vi "for_debugs.vi"() -> ()   [LabVIEW 2015]
uses:
  convertors/typedefs/BSONelement.ctl
  convertors/typedefs/dataType.ctl
  data_cluster.ctl
  convertors/typedefs/binaryData_cluster.ctl
  convertors/typedefs/arraySettings_cluster.ctl
  <vilib>/addons/_JKI.lib/Serialization/JSON/JKI JSON Serialization.lvlib
  convertors/BSON_convertors_Library.lvlib
panel:
  out "source data":T1={"int1"=1, "int2"=2, "SS1"={"int11"=11, "int22"=22}, "SS2"={"int33"=33, "int44"=44, "LLL"={"int1"=1, "int2"=2, "int11"=11, "int22"=22}}, "dblArray"=[111.1, 112.2, 113.3, 114.0, 115.0, 116.0, 117.0, 118.0, 119.0, 120.0], "stringData"="", "U64Array"=[5555, 5556, 5557, 5558, 5559, 5560, 5561]}
  in  "Tab Control":T2(tab)
  out "JSON String":string
  out "to_BSON_error out":errorcluster
  out "BSONdocArrayAsBin":u8[](array[numeric]) format="%02x"
  out "BSONdocArrayAsArray":u8[](array[numeric]) format="%02x"
  out "to_BSON_error out 2":errorcluster
  out "arrayOfElements_hiLVL_BinData":T3[](array[typedef])
  out "arrayOfElements_first_step":T3[](array[typedef])
  out "big cluster value":T3[](array[typedef])
  out "lvl2_cluster":T3[](array[typedef])
  out "arrayOfElements_hiLVL_arrays":T3[](array[typedef])
  out "diff names (error)":T5
  out "bindata error 5001 (error)":errorcluster
  out "diff names with array (error)":T5
  out "array error 5001 (error)":errorcluster
  out "strictData from bin":T1
  out "strictData error out1":errorcluster
  out "strictData from array":T1
  out "strictData error out2":errorcluster
  out "more elements from array":T6={"int1"=1, "int2"=2, "SS1"={"int11"=11, "int22"=22}, "SS2"={"int33"=33, "int44"=44, "LLL"={"int1"=1, "int2"=2, "int11"=11, "int22"=22}}, "dblArray"=[111.0, 112.0, 113.0, 114.0, 115.0, 116.0, 117.0, 118.0, 119.0, 120.0], "U64Array"=[5555, 5556, 5557, 5558, 5559, 5560, 5561], "int88"=0, "stringData"=""}
  out "more elements from byte error out":errorcluster
  out "more elements from array error out":errorcluster
  out "more elements from bite":T6={"int1"=1, "int2"=2, "SS1"={"int11"=11, "int22"=22}, "SS2"={"int33"=33, "int44"=44, "LLL"={"int1"=1, "int2"=2, "int11"=11, "int22"=22}}, "dblArray"=[111.0, 112.0, 113.0, 114.0, 115.0, 116.0, 117.0, 118.0, 119.0, 120.0], "U64Array"=[5555, 5556, 5557, 5558, 5559, 5560, 5561], "int88"=0, "stringData"=""}
  out "Less elements from array 2":T7={"int1"=1, "int2"=2, "SS1"={"int11"=11, "int22"=22}, "SS2"={"int33"=33, "int44"=44, "LLL"={"int1"=1, "int2"=2, "int11"=11, "int22"=22}}, "dblArray"=[5555.0, 5556.0, 5557.0, 5558.0, 5559.0, 5560.0, 5561.0], "stringData"=""}
  out "Less elements from binary as binArray error out":errorcluster
  out "Less elements from binary as binArray":T8={"int1"=1, "int2"=2, "SS1"={"int11"=11, "int22"=22}, "SS2"={"int33"=33, "int44"=44, "LLL"={"int1"=1, "int2"=2, "int11"=11, "int22"=22}}, "U64Array"=[], "stringData"=""}
  out "Less elements from binary as binCluster error out":errorcluster
  out "Less elements from binary as binCluster":T10={"int1"=1, "int2"=2, "SS1"={"int11"=11, "int22"=22}, "SS2"={"int33"=33, "int44"=44, "LLL"={"int1"=1, "int2"=2, "int11"=11, "int22"=22}}, "dblArray"={"subType"=0, "byteArray"=[]}, "stringData"=""}
  out "Less elements from array":T11={"int1"=1, "int2"=2, "SS1"={"int11"=11, "int22"=22}, "SS2"={"int33"=33, "int44"=44, "LLL"={"int1"=1, "int2"=2, "int11"=11, "int22"=22}}, "U64Array"=[5555, 5556, 5557, 5558, 5559, 5560, 5561], "stringData"=""}
  out "Less elements from binary error out":errorcluster
  out "Less elements from array error out":errorcluster
  out "Less elements from binary":T7={"int1"=1, "int2"=2, "SS1"={"int11"=11, "int22"=22}, "SS2"={"int33"=33, "int44"=44, "LLL"={"int1"=1, "int2"=2, "int11"=11, "int22"=22}}, "dblArray"=[111.0, 112.0, 113.0, 114.0, 115.0, 116.0, 117.0, 118.0, 119.0, 120.0], "stringData"=""}
  out "Less elements from array error out 2":errorcluster
  # "This clusters have \"illegal\" elements for strict conversion"
  # "These clusters are exactly the same as in the package"
  # "These clusters have \"extra\" elements.\nOnly those that are in the package are filled"
  # "This clusters have fewer elements.\nOnly those that are present are filled. Excess data from the package is discarded"
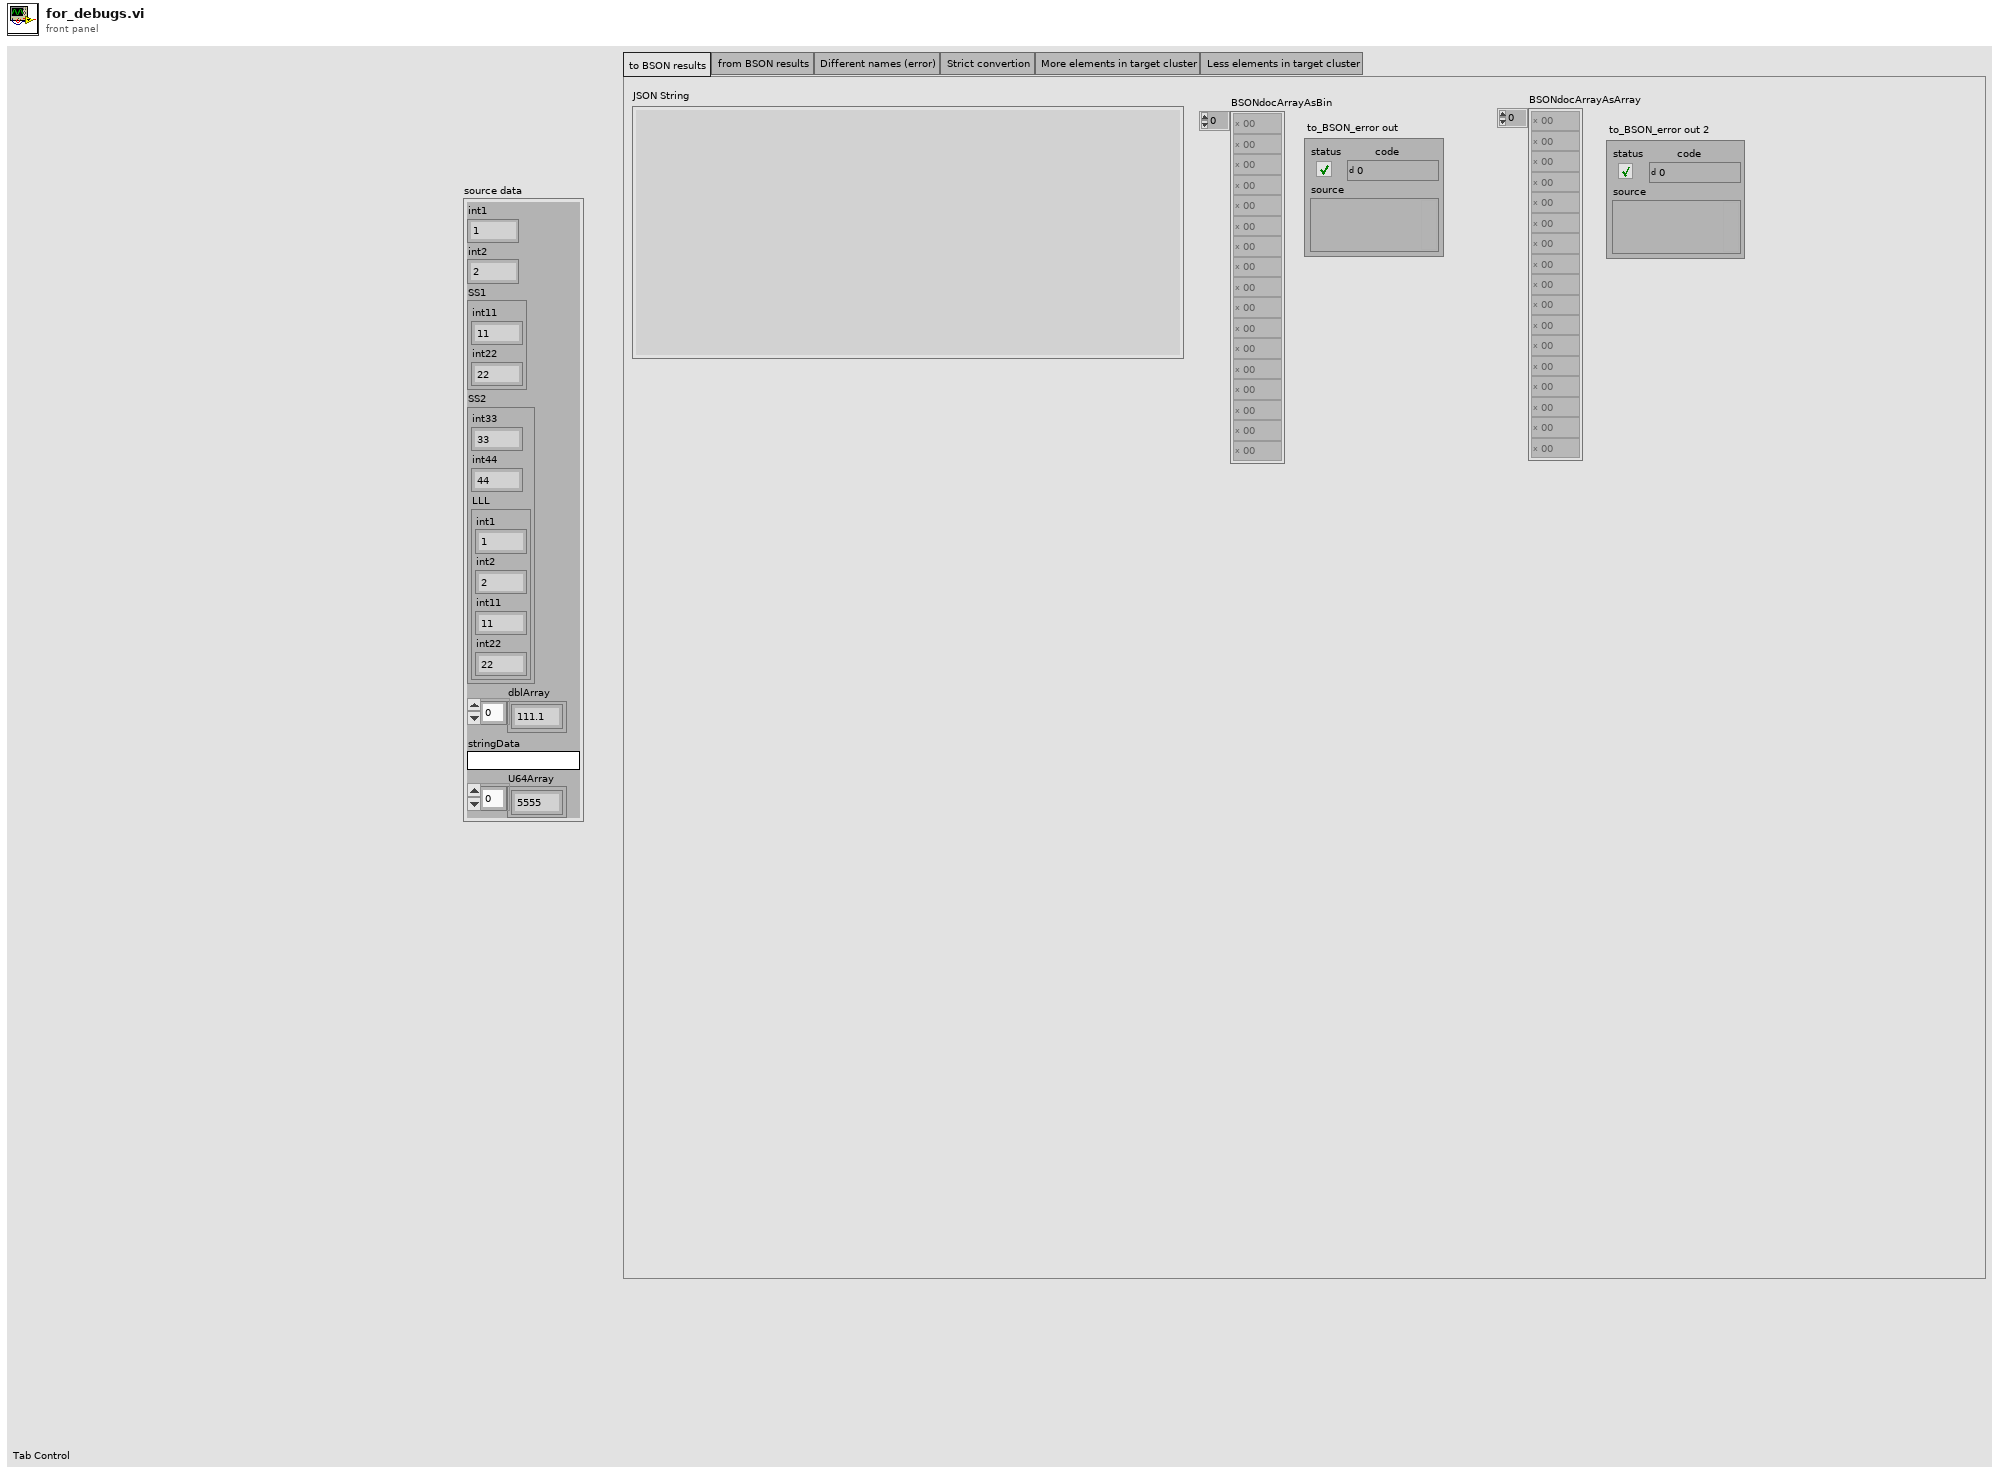
[diagram p1: front panel]
types:
  T1 = typedef "data_cluster.ctl" = cluster{"int1":i32, "int2":i32, "SS1":cluster{"int11":i32, "int22":i32}, "SS2":cluster{"int33":i32, "int44":i32, "LLL":cluster{"int1":i32, "int2":i32, "int11":i32, "int22":i32}}, "dblArray":dbl[], "stringData":string, "U64Array":u64[]}
  T2 = enum32{"to BSON results", "from BSON results", "Different names (error)", "Strict convertion", "More elements in target cluster", "Less elements in target cluster"}
  T3 = typedef "BSON_convertors_Library.lvlib/BSONelement.ctl" = cluster{"dataType":T4, "name":string, "value":variant}
  T4 = typedef "BSON_convertors_Library.lvlib/dataType.ctl" = enum8{"empty(terminator)", "double", "string", "document", "array", "binary", "Deprecated(Undefined)", "ObjectId", "boolean", "UTC datetime", "Null value", "cstring", "Deprecated(DBPointer)", "JavaScript", "Deprecated(Symbol)", "code_w_s", "int32", "uint64", "int64", "ext (decimal128)", "Min key", "Max key"}
  T5 = cluster{"int1":i32, "int2":i32, "SS1":cluster{"int11":i32, "int22":i32}, "SS2":cluster{"int3333":i32, "int44":i32, "LLL":cluster{"int1":i32, "int2":i32, "int11":i32, "int22":i32}}}
  T6 = cluster{"int1":i32, "int2":i32, "SS1":cluster{"int11":i32, "int22":i32}, "SS2":cluster{"int33":i32, "int44":i32, "LLL":cluster{"int1":i32, "int2":i32, "int11":i32, "int22":i32}}, "dblArray":dbl[], "U64Array":u64[], "int88":i32, "stringData":string}
  T7 = cluster{"int1":i32, "int2":i32, "SS1":cluster{"int11":i32, "int22":i32}, "SS2":cluster{"int33":i32, "int44":i32, "LLL":cluster{"int1":i32, "int2":i32, "int11":i32, "int22":i32}}, "dblArray":dbl[], "stringData":string}
  T8 = cluster{"int1":i32, "int2":i32, "SS1":cluster{"int11":i32, "int22":i32}, "SS2":cluster{"int33":i32, "int44":i32, "LLL":cluster{"int1":i32, "int2":i32, "int11":i32, "int22":i32}}, "U64Array":u8[], "stringData":string}
  T9 = typedef "BSON_convertors_Library.lvlib/binaryData_cluster.ctl" = cluster{"subType":u8, "byteArray":u8[]}
  T10 = cluster{"int1":i32, "int2":i32, "SS1":cluster{"int11":i32, "int22":i32}, "SS2":cluster{"int33":i32, "int44":i32, "LLL":cluster{"int1":i32, "int2":i32, "int11":i32, "int22":i32}}, "dblArray":T9, "stringData":string}
  T11 = cluster{"int1":i32, "int2":i32, "SS1":cluster{"int11":i32, "int22":i32}, "SS2":cluster{"int33":i32, "int44":i32, "LLL":cluster{"int1":i32, "int2":i32, "int11":i32, "int22":i32}}, "U64Array":u64[], "stringData":string}
  T12 = typedef "BSON_convertors_Library.lvlib/arraySettings_cluster.ctl" = cluster{"arrayAsBinData":bool, "binDataSubType":u8, "little-endian":bool}
  T13 = enum16{"open", "replace", "create", "open or create", "replace or create", "replace or create with confirmation"}
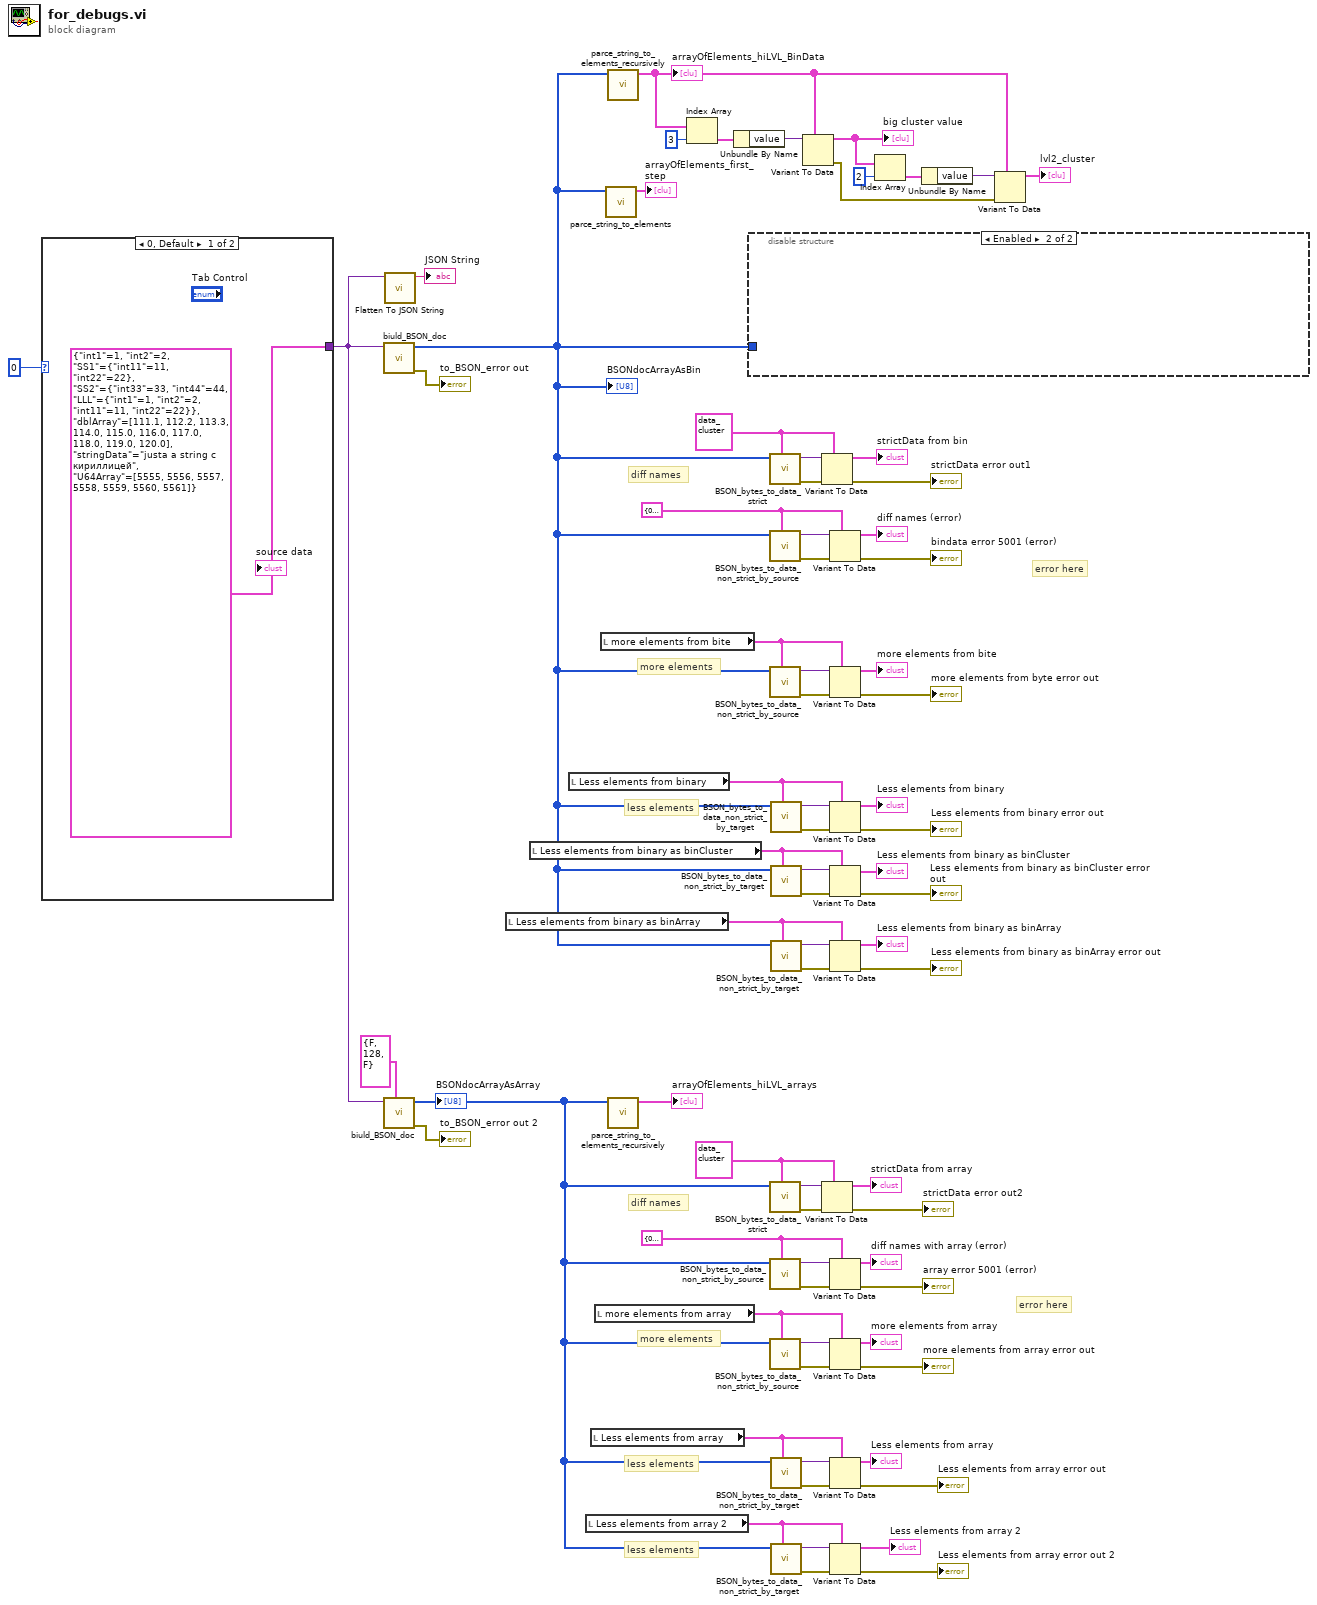
[diagram p0: block diagram]
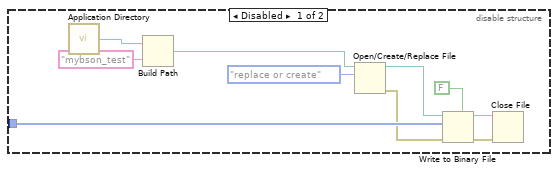
[diagram p2: hidden frame]
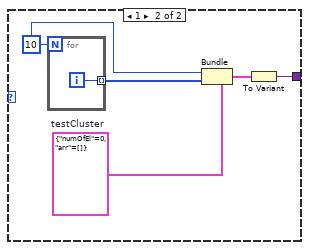
[diagram p3: hidden frame]
diagram:
  w45 = T1 {"int1"=0, "int2"=0, "SS1"={"int11"=0, "int22"=0}, "SS2"={"int33"=0, "int44"=0, "LLL"={"int1"=0, "int2"=0, "int11"=0, "int22"=0}}, "dblArray"=[], "stringData"="", "U64Array"=[]} ("LLL")
  w43 = T5 {"int1"=0, "int2"=0, "SS1"={"int11"=0, "int22"=0}, "SS2"={"int3333"=0, "int44"=0, "LLL"={"int1"=0, "int2"=0, "int11"=0, "int22"=0}}}
  w51 = T1 {"int1"=0, "int2"=0, "SS1"={"int11"=0, "int22"=0}, "SS2"={"int33"=0, "int44"=0, "LLL"={"int1"=0, "int2"=0, "int11"=0, "int22"=0}}, "dblArray"=[], "stringData"="", "U64Array"=[]} ("LLL")
  w53 = T5 {"int1"=0, "int2"=0, "SS1"={"int11"=0, "int22"=0}, "SS2"={"int3333"=0, "int44"=0, "LLL"={"int1"=0, "int2"=0, "int11"=0, "int22"=0}}}
  # "less elements"
  # "more elements"
  # "less elements"
  # "less elements"
  # "error here"
  # "diff names"
  # "more elements"
  # "error here"
  # "diff names"
  n1 = case shown="0, Default" 0 {
    tunnel: [w76 w78] -> w61
    frame 0, Default {
      w76 = T1 {"int1"=1, "int2"=2, "SS1"={"int11"=11, "int22"=22}, "SS2"={"int33"=33, "int44"=44, "LLL"={"int1"=1, "int2"=2, "int11"=11, "int22"=22}}, "dblArray"=[111.1, 112.2, 113.3, 114.0, 115.0, 116.0, 117.0, 118.0, 119.0, 120.0], "stringData"="justa a string с кириллицей", "U64Array"=[5555, 5556, 5557, 5558, 5559, 5560, 5561]} ("output cluster")
      "source data" <- w76
    }
    frame 1 {
      w77 = cluster{"numOfEl":i32, "arr":u8[]} {"numOfEl"=0, "arr"=[]}  # testCluster
      w80 = 10
      n2 = for {
        N: w80 -> [_]
        tunnel: [w82] -> w81 mode=indexing
        i -> [w82]
      }
      n3 = Bundle(cluster=w77, "numOfEl"=w80, "arr"=w81) -> (w79:cluster{"numOfEl":i32, "arr":u8[]})
      n4 = To Variant(anything=w79) -> (Variant=w78:variant)
    }
  }
  n5 = call "biuld_BSON_doc.vi"("data"=w61) -> ("error out"=→"to_BSON_error out":errorcluster, "BSONdoc"=w60:u8[])  [unwired: 9 in]
  "BSONdocArrayAsBin" <- w60
  n6 = call "biuld_BSON_doc.vi"("arrayAsBin(T, x80, T)"=T12 {"arrayAsBinData"=FALSE, "binDataSubType"=128, "little-endian"=FALSE} ("arrayAsBin(T, x80)"), "data"=w61) -> ("error out"=→"to_BSON_error out 2":errorcluster, "BSONdoc"=w22:u8[])  [unwired: 8 in]
  "BSONdocArrayAsArray" <- w22
  n7 = call <vilib>:"Flatten To JSON String.vi"("Variant"=w61) -> ("JSON String"=→"JSON String":string)  [unwired: 9 in, 1 out]
  n8 = local read "Less elements from binary as binArray"() -> (w4:T8)
  n9 = local read "Less elements from binary as binCluster"() -> (w5:T10)
  n10 = local read "Less elements from binary"() -> (w12:T7)
  n11 = local read "Less elements from array 2"() -> (w26:T7)
  n12 = local read "Less elements from array"() -> (w27:T11)
  n13 = local read "more elements from array"() -> (w32:T6)
  n14 = local read "more elements from bite"() -> (w16:T6)
  n15 = call "parce_string_to_elements.vi"("BSONbytes"=w60) -> ("arrayOfElements"=→"arrayOfElements_first_step":T3[])  [unwired: 8 in, 2 out]
  n16 = call "parce_string_to_elements_recursively.vi"("BSONdoc"=w60) -> ("arrayOfElements"=w66:T3[])  [unwired: 9 in, 1 out]
  "arrayOfElements_hiLVL_BinData" <- w66
  n17 = call "parce_string_to_elements_recursively.vi"("BSONdoc"=w22) -> ("arrayOfElements"=→"arrayOfElements_hiLVL_arrays":T3[])  [unwired: 9 in, 1 out]
  n18 = Index Array(array=w66, index=3) -> (element=w72:T3)
  n19 = Unbundle By Name(w72) -> ("value"=w71:variant)
  n20 = disable-structure shown="Enabled" {
    disable-tunnel: w60 -> [w88 _]
    frame Disabled {
      n21 = call <vilib>:"Application Directory.vi"() -> ("Application Directory"=w84:path)
      n22 = Build Path(base path=w84, name or relative path="mybson_test") -> (appended path=w83:path)
      n23 = Open/Create/Replace File(file path (use dialog)=w83, operation (0:open)=T13."replace or create") -> (refnum out=w90:refnum<file>, error out=w87:errorcluster)  [unwired: 4 in, 1 out]
      n24 = Write to Binary File(file (use dialog)=w90, data=w88, error in=w87, 5:FALSE ("prepend array or string size? (T)")) -> (refnum out=w89:refnum<file>, error out=w86:errorcluster)  [unwired: 2 in, 1 out]
      n25 = Close File(refnum=w89, error in=w86) -> ()  [unwired: 2 out]
    }
    frame Enabled {
    }
  }
  n26 = call "BSON_bytes_to_data_strict.vi"("dataType"=w51, "BSONbytes"=w60) -> ("error out"=w58:errorcluster, "result"=w59:variant)  [unwired: 8 in]
  n27 = call "BSON_bytes_to_data_non_strict_by_source.vi"("dataType"=w53, "BSONbytes"=w60) -> ("error out"=w56:errorcluster, "result"=w55:variant)  [unwired: 8 in]
  n28 = call "BSON_bytes_to_data_non_strict_by_source.vi"("dataType"=w16, "BSONbytes"=w60) -> ("error out"=w19:errorcluster, "result"=w20:variant)  [unwired: 8 in]
  n29 = call "BSON_bytes_to_data_strict.vi"("dataType"=w45, "BSONbytes"=w22) -> ("error out"=w38:errorcluster, "result"=w37:variant)  [unwired: 8 in]
  n30 = call "BSON_bytes_to_data_non_strict_by_source.vi"("dataType"=w43, "BSONbytes"=w22) -> ("error out"=w40:errorcluster, "result"=w41:variant)  [unwired: 8 in]
  n31 = call "BSON_bytes_to_data_non_strict_by_source.vi"("dataType"=w32, "BSONbytes"=w22) -> ("error out"=w35:errorcluster, "result"=w34:variant)  [unwired: 8 in]
  n32 = call "BSON_bytes_to_data_non_strict_by_target.vi"("dataType"=w12, "BSONbytes"=w60) -> ("error out"=w14:errorcluster, "result"=w15:variant)  [unwired: 8 in]
  n33 = call "BSON_bytes_to_data_non_strict_by_target.vi"("dataType"=w5, "BSONbytes"=w60) -> ("error out"=w10:errorcluster, "result"=w9:variant)  [unwired: 8 in]
  n34 = call "BSON_bytes_to_data_non_strict_by_target.vi"("dataType"=w4, "BSONbytes"=w60) -> ("error out"=w7:errorcluster, "result"=w8:variant)  [unwired: 8 in]
  n35 = call "BSON_bytes_to_data_non_strict_by_target.vi"("dataType"=w27, "BSONbytes"=w22) -> ("error out"=w31:errorcluster, "result"=w30:variant)  [unwired: 8 in]
  n36 = call "BSON_bytes_to_data_non_strict_by_target.vi"("dataType"=w26, "BSONbytes"=w22) -> ("error out"=w23:errorcluster, "result"=w24:variant)  [unwired: 8 in]
  n37 = Variant To Data(type=w66, Variant=w71) -> (data=w68:T3[], error out=w64:errorcluster)  [unwired: 1 in]
  "big cluster value" <- w68
  n38 = Variant To Data(error in=w58, type=w51, Variant=w59) -> (data=→"strictData from bin":T1, error out=→"strictData error out1":errorcluster)
  n39 = Variant To Data(error in=w38, type=w45, Variant=w37) -> (data=→"strictData from array":T1, error out=→"strictData error out2":errorcluster)
  n40 = Variant To Data(error in=w56, type=w53, Variant=w55) -> (data=→"diff names (error)":T5, error out=→"bindata error 5001 (error)":errorcluster)
  n41 = Variant To Data(error in=w19, type=w16, Variant=w20) -> (data=→"more elements from bite":T6, error out=→"more elements from byte error out":errorcluster)
  n42 = Variant To Data(error in=w14, type=w12, Variant=w15) -> (data=→"Less elements from binary":T7, error out=→"Less elements from binary error out":errorcluster)
  n43 = Variant To Data(error in=w10, type=w5, Variant=w9) -> (data=→"Less elements from binary as binCluster":T10, error out=→"Less elements from binary as binCluster error out":errorcluster)
  n44 = Variant To Data(error in=w7, type=w4, Variant=w8) -> (data=→"Less elements from binary as binArray":T8, error out=→"Less elements from binary as binArray error out":errorcluster)
  n45 = Variant To Data(error in=w40, type=w43, Variant=w41) -> (data=→"diff names with array (error)":T5, error out=→"array error 5001 (error)":errorcluster)
  n46 = Variant To Data(error in=w35, type=w32, Variant=w34) -> (data=→"more elements from array":T6, error out=→"more elements from array error out":errorcluster)
  n47 = Variant To Data(error in=w31, type=w27, Variant=w30) -> (data=→"Less elements from array":T11, error out=→"Less elements from array error out":errorcluster)
  n48 = Variant To Data(error in=w23, type=w26, Variant=w24) -> (data=→"Less elements from array 2":T7, error out=→"Less elements from array error out 2":errorcluster)
  n49 = Index Array(array=w68, index=2) -> (element=w70:T3)
  n50 = Unbundle By Name(w70) -> ("value"=w67:variant)
  n51 = Variant To Data(error in=w64, type=w66, Variant=w67) -> (data=→"lvl2_cluster":T3[])  [unwired: 1 out]
